vi "Gateway.vi"(0 "setMeasurement":bool, 1 "startClock":bool, 2 "startCollection":bool, 3 "stopCollection":bool, 4 "setTermination":bool, 5 "ClockFrequency":dbl=1.0 min=1.0 max=2500000.0, 6 "filename":string) -> (12 "nameout":string, 14 "stateMeasurement":bool, 15 "stateClock":bool, 16 "ErrorDescription":string, 17 "stateCollection":bool, 19 "stateError":bool)   [LabVIEW 2009]
panel:
  in  "stopClock":bool
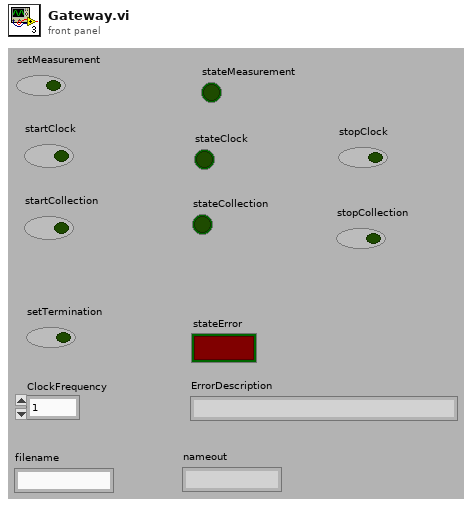
[diagram p1: front panel]
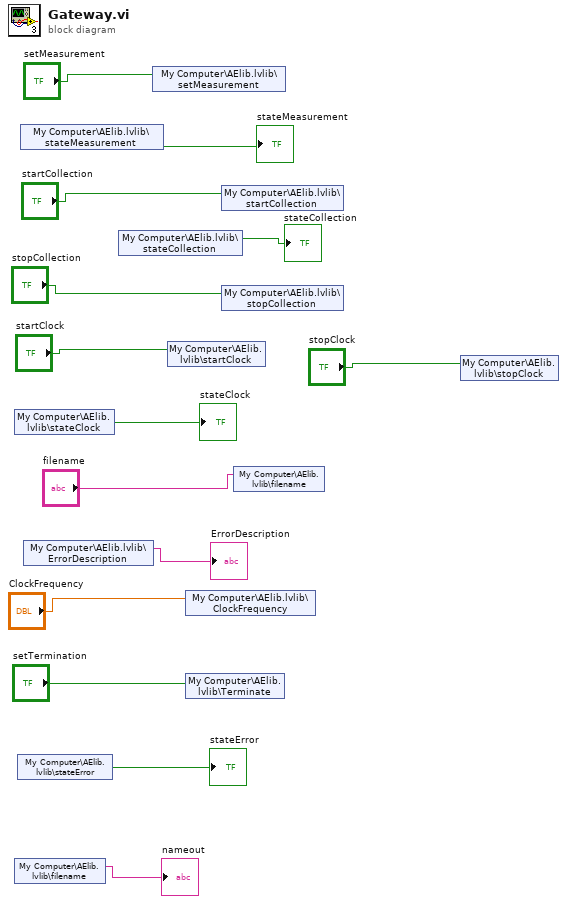
[diagram p0: block diagram]
diagram:
  n1 = shared-variable "My Computer\\AElib.lvlib\\stateClock"() -> (→"stateClock":bool)  [unwired: 1 in, 1 out]
  n2 = shared-variable "My Computer\\AElib.lvlib\\filename"() -> (→"nameout":string)  [unwired: 1 in, 1 out]
  n3 = shared-variable "My Computer\\AElib.lvlib\\stateError"() -> (→"stateError":bool)  [unwired: 1 in, 1 out]
  n4 = shared-variable "My Computer\\AElib.lvlib\\stateMeasurement"() -> (→"stateMeasurement":bool)  [unwired: 1 in, 1 out]
  n5 = shared-variable "My Computer\\AElib.lvlib\\ErrorDescription"() -> (→"ErrorDescription":string)  [unwired: 1 in, 1 out]
  n6 = shared-variable "My Computer\\AElib.lvlib\\stateCollection"() -> (→"stateCollection":bool)  [unwired: 1 in, 1 out]
  n7 = shared-variable "My Computer\\AElib.lvlib\\setMeasurement"("setMeasurement") -> ()  [unwired: 1 in, 1 out]
  n8 = shared-variable "My Computer\\AElib.lvlib\\startClock"("startClock") -> ()  [unwired: 1 in, 1 out]
  n9 = shared-variable "My Computer\\AElib.lvlib\\ClockFrequency"("ClockFrequency") -> ()  [unwired: 1 in, 1 out]
  n10 = shared-variable "My Computer\\AElib.lvlib\\Terminate"("setTermination") -> ()  [unwired: 1 in, 1 out]
  n11 = shared-variable "My Computer\\AElib.lvlib\\startCollection"("startCollection") -> ()  [unwired: 1 in, 1 out]
  n12 = shared-variable "My Computer\\AElib.lvlib\\stopCollection"("stopCollection") -> ()  [unwired: 1 in, 1 out]
  n13 = shared-variable "My Computer\\AElib.lvlib\\filename"("filename") -> ()  [unwired: 1 in, 1 out]
  n14 = shared-variable "My Computer\\AElib.lvlib\\stopClock"("stopClock") -> ()  [unwired: 1 in, 1 out]
